vi "Prompts_for_User.vi"   [LabVIEW 2017]
uses:
  1be5debe-3b1a-4dec-b588-72e4d14eac37.vi
  fe4dd19f-7f62-4b99-b512-7902f5b770d3.vi
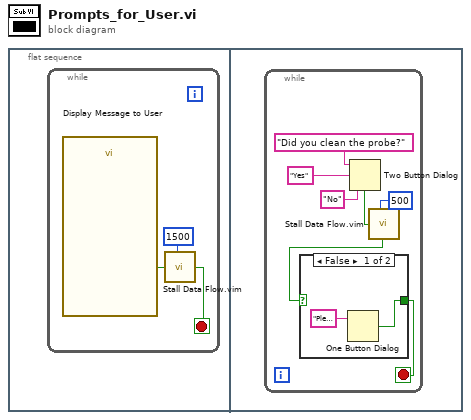
[diagram p0: block diagram]
diagram:
  n1 = flat-sequence {
    frame #0 {
      n2 = while {
        stop <- w1 stop-if-true
        n3 = call "Display Message to User"() -> ("Continue"=w2:bool)  [unwired: 10 in, 1 out]
        n4 = call "Stall Data Flow.vim"("value in"=w2, "milliseconds to wait"=1500) -> ("value out"=w1:bool)  [unwired: 1 out]
      }
    }
    frame #1 {
      n5 = while {
        stop <- w4 stop-if-true
        n6 = Two Button Dialog(message="Did you clean the probe?", 1:"No", 2:"Yes") -> (T button?=w6:bool)
        n7 = call "Stall Data Flow.vim"("value in"=w6, "milliseconds to wait"=500) -> ("value out"=w5:bool)  [unwired: 1 out]
        n8 = case shown="False" w5 {
          selector: w5 -> [_ w13]
          tunnel: [w11 w13] -> w4
          frame False {
            n9 = One Button Dialog(message="Please clean probe head with wipe before proceeding") -> (true=w11:bool)  [unwired: 1 in]
          }
          frame True {
          }
        }
      }
    }
  }
